vi "Photo Isp Get Luminous Flux.vi"(8 "error in (no error)":errorcluster, 9 "a_ispsurfacecm2":dbl, 10 "a_CIEResolution":u8, 11 "a_data":dbl[](array[numeric])) -> (0 "error out":errorcluster, 2 "function return":i16, 3 "a_data out":dbl[](array[numeric]), 5 "a_Lumen out":dbl)   [LabVIEW 2013, in "AvaSpec.lvlib" / "AVSirrad.lvlib"]
doc: "DLL_API short int __stdcall Photo_IspGetLuminousFlux\n(\n DataType *a_data,\n unsigned char a_CIEResolution,\n double a_ispsurfacecm2,\n double *a_Lumen\n);"
uses:
  AVSirrad.lvlib
  AVSirrad.dll
panel:
  in  "a_Lumen":dbl
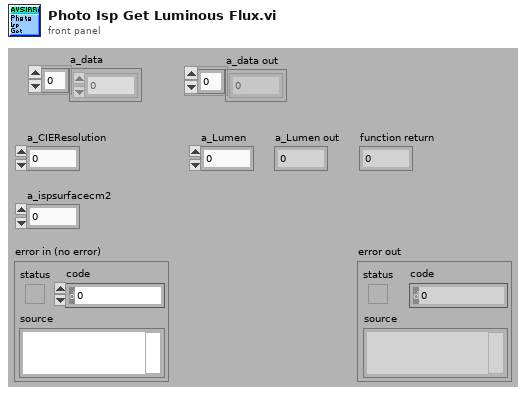
[diagram p1: front panel]
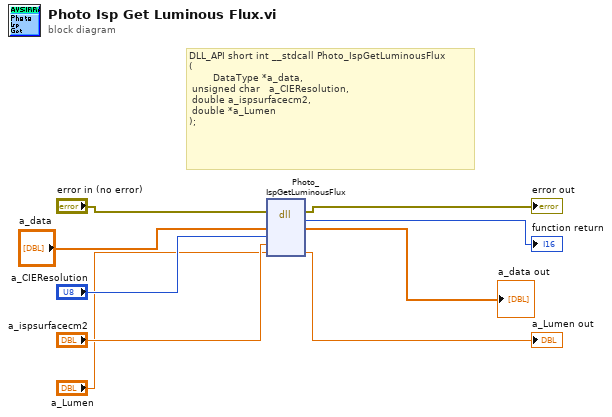
[diagram p0: block diagram]
diagram:
  # "DLL_API short int __stdcall Photo_IspGetLuminousFlux\n(\n        DataType *a_data,\n\tunsigned char   a_CIEResolution,\n\tdouble a_ispsurfacecm2,\n\tdouble *a_Lumen\n);"
  n1 = dll-call lib="C:/Users/dhstuart/Dropbox/CLTC/avantesSpectrometer/Libraries/IRRAD-DLL/AVSirrad.*" fn="Photo_IspGetLuminousFlux"(error in="error in (no error)", "a_data"="a_data", "a_CIEResolution"="a_CIEResolution", "a_ispsurfacecm2"="a_ispsurfacecm2", "a_Lumen"="a_Lumen") -> (error out=→"error out":errorcluster, "return type"=→"function return":i16, "a_data"=→"a_data out":dbl[], "a_Lumen"=→"a_Lumen out":dbl)  [unwired: 4 in, 1 out]
